vi "Lighthouse Monitoring And Control System.vi"() -> ()   [LabVIEW 2012]
uses:
  <vilib>/DAQmx/create/channels.llb/DAQmx Create Channel (AI-Voltage-Basic).vi
  <vilib>/DAQmx/read.llb/DAQmx Read (Analog DBL 1Chan 1Samp).vi
panel:
  in  "physical channels":tag
  out "Light Intensity Meter":dbl(knob) scale=0.0..10.0
  in  "On / Off":bool
  in  "?":bool
  # "Lighthouse Monitoring & Control System"
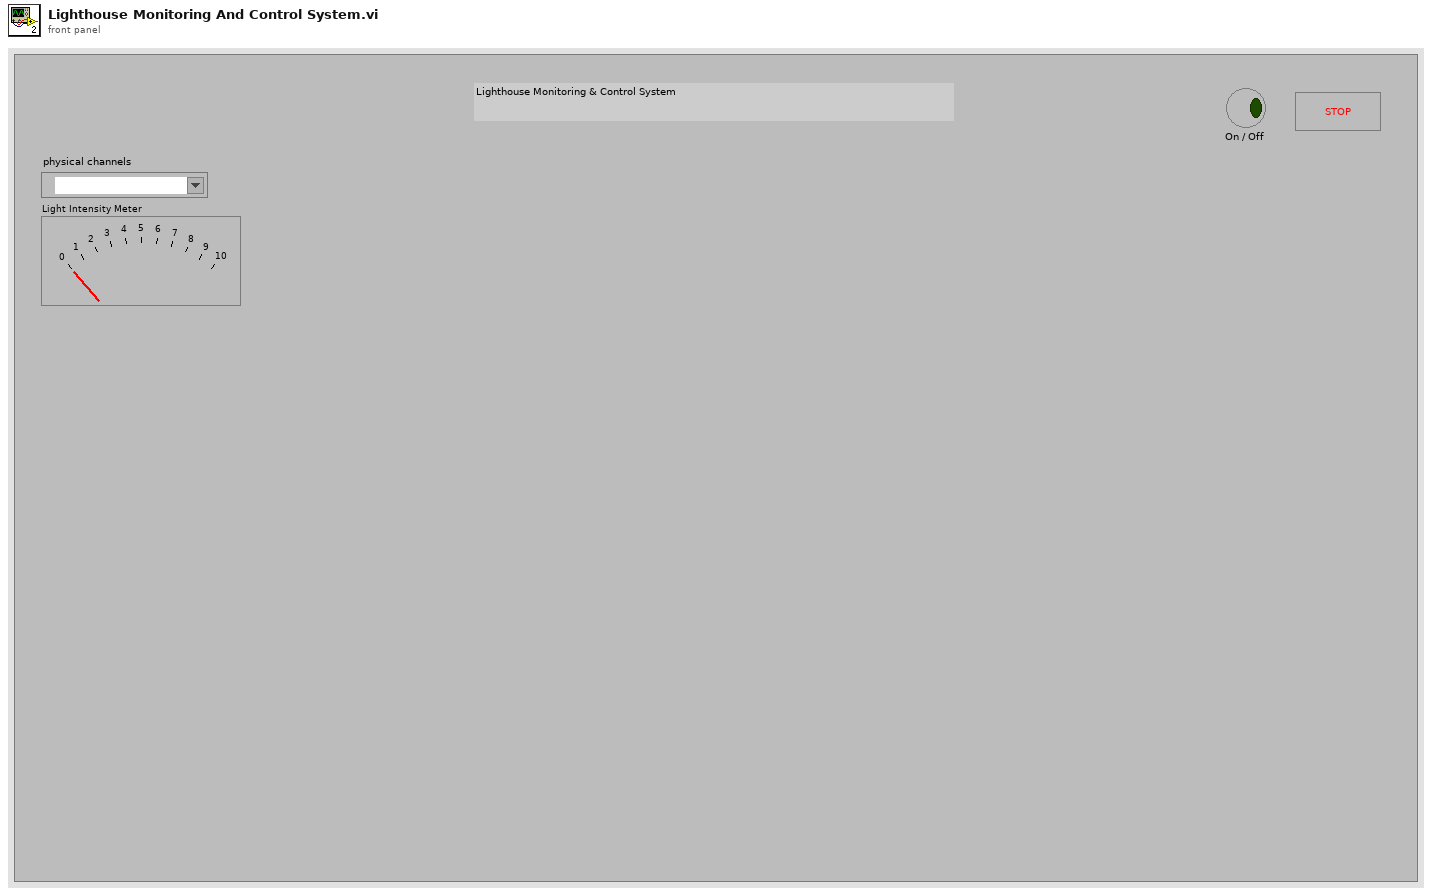
[diagram p1: front panel]
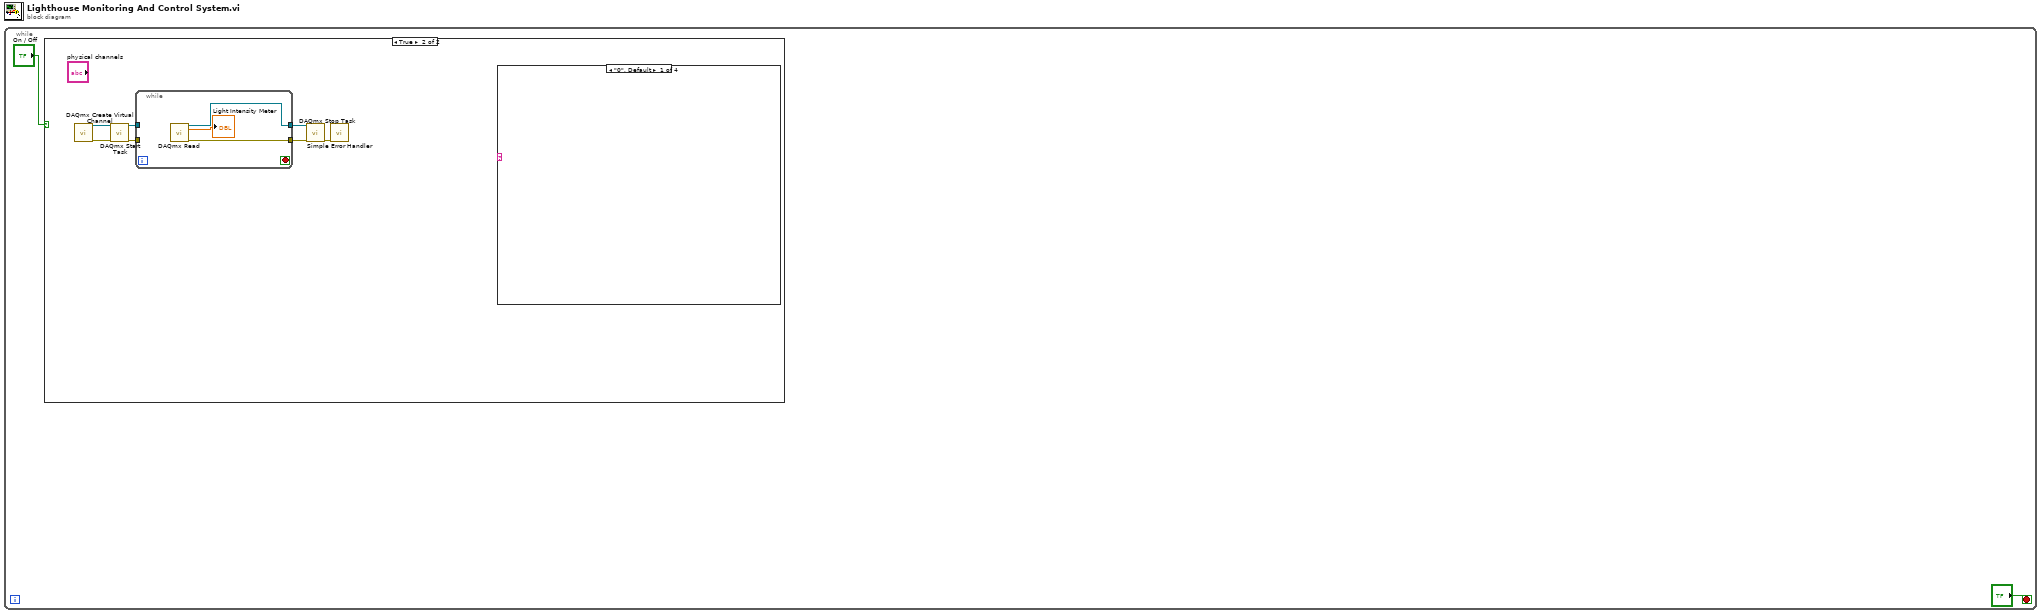
[diagram p0: block diagram]
diagram:
  n1 = while {
    stop <- "?" stop-if-true
    n2 = case shown="True" "On / Off" {
      frame False {
      }
      frame True {
        n3 = call-poly <vilib>:"DAQmx Create Virtual Channel.vi"() -> ("task out"=w8:refnum<k21>, "error out"=w9:errorcluster)  [unwired: 14 in]
        n4 = call <vilib>:"DAQmx Start Task.vi"("task/channels in"=w8, "error in"=w9) -> ("task out"=w6:refnum<k21>, "error out"=w7:errorcluster)  [unwired: 12 in]
        n5 = while {
          tunnel: w7 -> [_]
          tunnel: w6 -> [_]
          tunnel: [w12] -> w5
          tunnel: [w11] -> w3
          stop <- _ stop-if-true
          n6 = call-poly <vilib>:"DAQmx Read.vi"() -> ("task out"=w11:refnum<k21>, "data"=→"Light Intensity Meter":dbl, "error out"=w12:errorcluster)  [unwired: 13 in]
        }
        n7 = call <vilib>:"DAQmx Stop Task.vi"("task/channels in"=w3, "error in"=w5) -> ("error out"=w4:errorcluster)  [unwired: 12 in, 1 out]
        n8 = call <vilib>:"Simple Error Handler.vi"("error in (no error)"=w4) -> ()  [unwired: 4 in, 5 out]
        n9 = case shown="\"0\", Default" {
          selector: _ -> [_ _ _ _]
          frame "0", Default {
          }
          frame "1".."2" {
          }
          frame "3".."4" {
          }
          frame "5" {
          }
        }
      }
    }
  }
